vi "realgas Soave 2.1.vi"(0 "Stoffmenge H2 [mol]":dbl, 1 "Stoffmenge CH4 [mol]":dbl, 2 "Stoffmenge C2H2 [mol]":dbl, 3 "Stoffmenge O2 [mol]":dbl, 4 "Stoffmenge N2 [mol]":dbl, 5 "T [K]":dbl, 8 "1. Befüllschritt":u16(ring) items=["H2", "CH4", "C2H2", "O2", "N2"], 9 "4. Befüllschritt":u16(ring) items=["H2", "CH4", "C2H2", "O2", "N2"], 10 "2. Befüllschritt":u16(ring) items=["H2", "CH4", "C2H2", "O2", "N2"], 11 "5. Befüllschritt":u16(ring) items=["H2", "CH4", "C2H2", "O2", "N2"], 12 "3. Befüllschritt":u16(ring) items=["H2", "CH4", "C2H2", "O2", "N2"]) -> (20 "Druck [bar]":ext[](array[numeric]))   [LabVIEW 2009]
uses:
  <vilib>/express/express arith-compare/Formula/XNode/ExpressFormulaBlockNode.xnode
  <vilib>/Analysis/NI_AALBase.lvlib
  <vilib>/Analysis/baseanly.llb/Real Outer Product.vi
  <vilib>/Analysis/baseanly.llb/Real Dot Product.vi
panel:
  in  "Stoffwerte der Gase":cluster{"Tabellenwerte":dbl[]}[](array[cluster])
  in  "Kammervolumen [m^3]":dbl
  # "Befüllreihenfolge"
  # "nach 1. Schritt"
  # "nach 2. Schritt"
  # "nach 3. Schritt"
  # "nach 4. Schritt"
  # "nach 5. Schritt"
  # "p,c [Pa]"
  # "Azentischer Wert"
  # "T,c [K]"
  # "H2"
  # "CH4"
  # "C2H2"
  # "O2"
  # "N2"
  # "CO2"
  # "H2O"
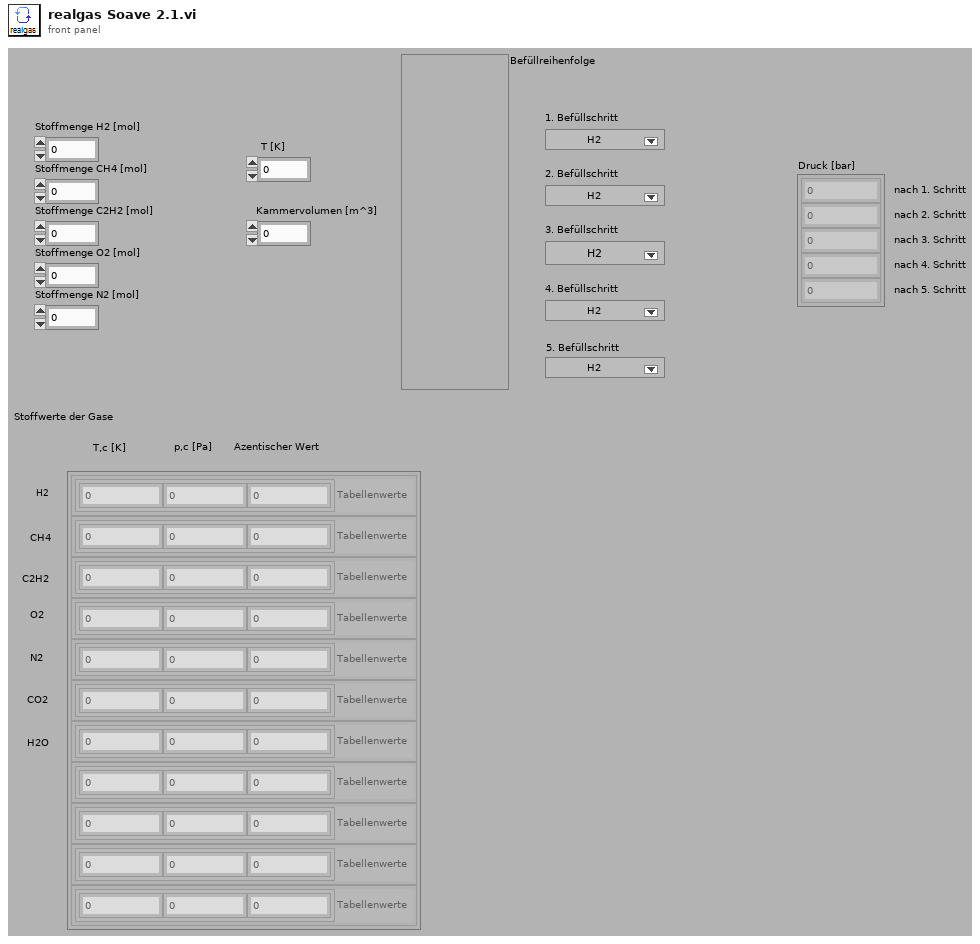
[diagram p1: front panel]
types:
  T1 = typedef "NI_Matrix.lvlib/RealMatrix.ctl" = dbl[][]
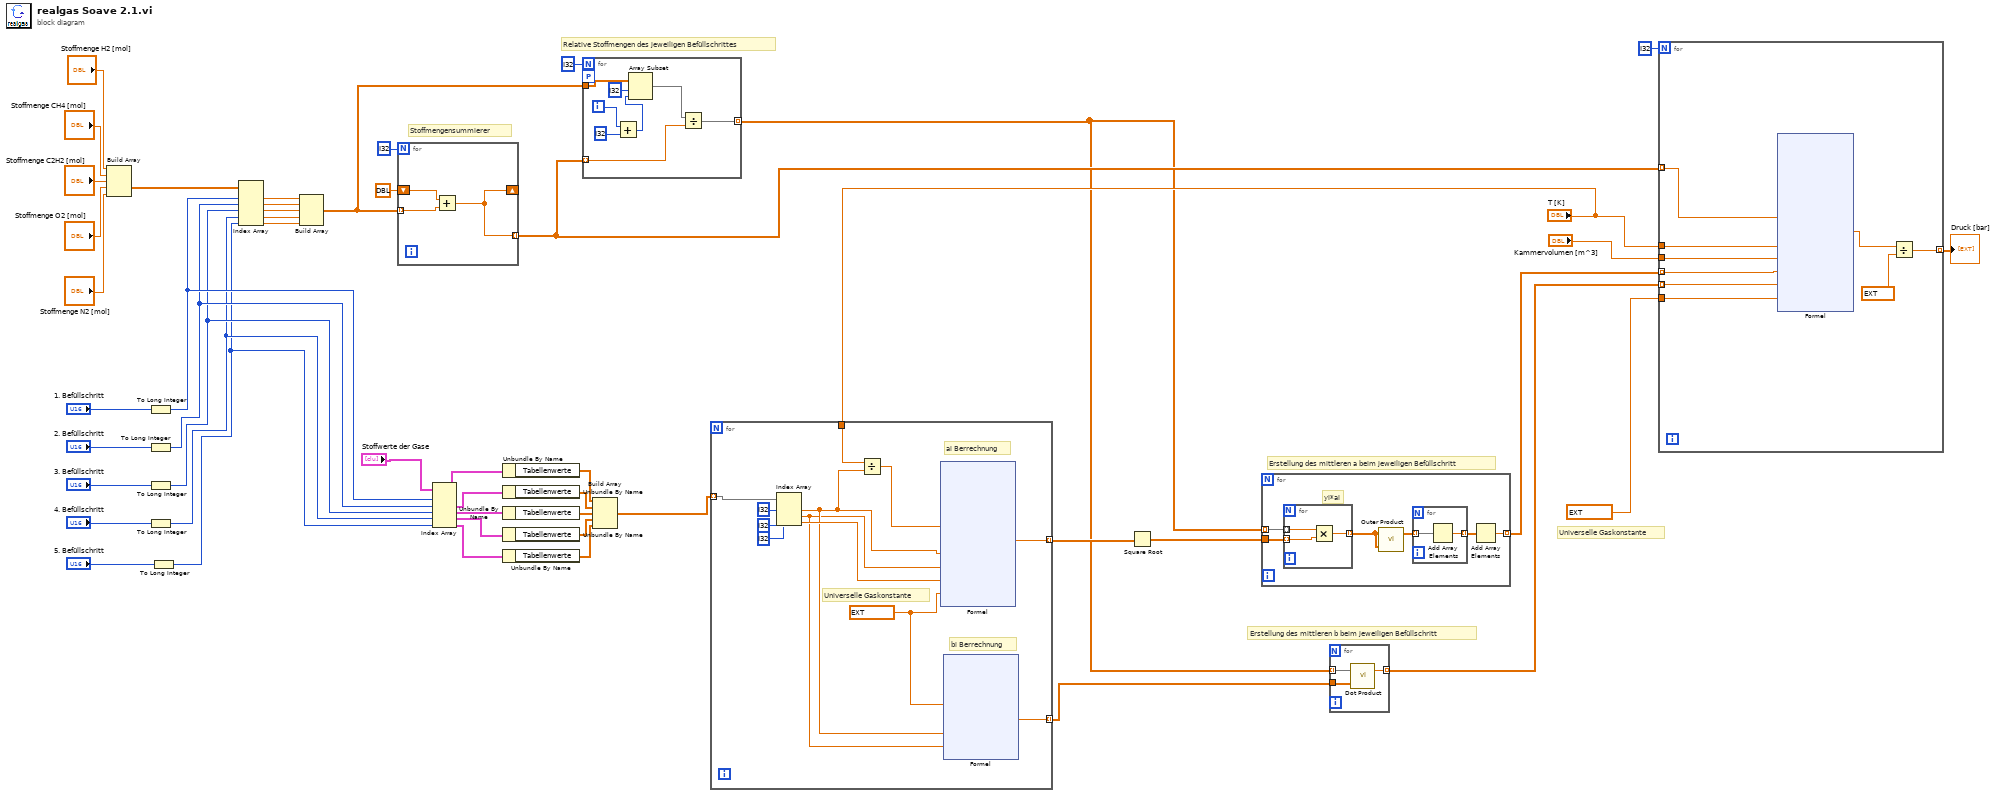
[diagram p0: block diagram]
diagram:
  # "Erstellung des mittleren b beim jeweiligen Befüllschritt"
  # "Relative Stoffmengen des jeweiligen Befüllschrittes"
  # "Stoffmengensummierer"
  # "Erstellung des mittleren a beim jeweiligen Befüllschritt"
  # "Universelle Gaskonstante"
  n1 = Build Array("Stoffmenge H2 [mol]", "Stoffmenge CH4 [mol]", "Stoffmenge C2H2 [mol]", "Stoffmenge O2 [mol]", "Stoffmenge N2 [mol]") -> (w39:dbl[])
  n2 = To Long Integer(number="1. Befüllschritt") -> (32bit integer=w26:i32)
  n3 = To Long Integer(number="2. Befüllschritt") -> (32bit integer=w25:i32)
  n4 = To Long Integer(number="3. Befüllschritt") -> (32bit integer=w24:i32)
  n5 = To Long Integer(number="4. Befüllschritt") -> (32bit integer=w23:i32)
  n6 = To Long Integer(number="5. Befüllschritt") -> (32bit integer=w22:i32)
  n7 = Index Array(array=w39, index #1=w26, index #2=w25, index #3=w24, index #4=w23, index #5=w22) -> (element #1=w38:dbl, element #2=w37:dbl, element #3=w36:dbl, element #4=w35:dbl, element #5=w34:dbl)
  n8 = Build Array(w38, w37, w36, w35, w34) -> (w10:dbl[])
  n9 = for {
    N: i32 ? -> [_]
    tunnel: w10 -> [w52] mode=indexing
    shift-right: [w50] -> _
    shift-left: dbl ? -> [w51]
    tunnel: [w50] -> w5 mode=indexing
    n10 = Add(x=w51, y=w52) -> (x+y=w50:dbl)
  }
  n11 = Index Array(array="Stoffwerte der Gase", index #1=w26, index #2=w25, index #3=w24, index #4=w23, index #5=w22) -> (element #1=w27:cluster{"Tabellenwerte":dbl[]}, element #2=w21:cluster{"Tabellenwerte":dbl[]}, element #3=w20:cluster{"Tabellenwerte":dbl[]}, element #4=w19:cluster{"Tabellenwerte":dbl[]}, element #5=w18:cluster{"Tabellenwerte":dbl[]})
  n12 = Unbundle By Name(w27) -> ("Tabellenwerte"=w17:dbl[])
  n13 = Unbundle By Name(w21) -> ("Tabellenwerte"=w16:dbl[])
  n14 = Unbundle By Name(w20) -> ("Tabellenwerte"=w15:dbl[])
  n15 = Unbundle By Name(w19) -> ("Tabellenwerte"=w14:dbl[])
  n16 = Unbundle By Name(w18) -> ("Tabellenwerte"=w13:dbl[])
  n17 = for {
    N: i32 ? -> [_]
    tunnel: w10 -> [w60]
    tunnel: w5 -> [w55] mode=indexing
    workers-P: _ -> [_]
    tunnel: [w53] -> w3 mode=indexing
    i -> [w58]
    n18 = Add(x=w58, y=i32 ?) -> (x+y=w56:i32)
    n19 = Array Subset(array=w60, index=i32 ? ("Index"), length=w56) -> (w54:dbl[])
    n20 = Divide(x=w54, y=w55) -> (x/y=w53:dbl[])
  }
  n21 = Build Array(w17, w16, w15, w14, w13) -> (w12:dbl[][])
  n22 = for {
    tunnel: w12 -> [w72] mode=indexing
    tunnel: "T [K]" -> [w68]
    tunnel: [w65] -> w7 mode=indexing
    tunnel: [w61] -> w4 mode=indexing
    w64 = ext ? ("Wert")
    # "bi Berrechnung"
    # "ai Berrechnung"
    # "Universelle Gaskonstante"
    n23 = Index Array(array=w72, index #1=i32 ? ("Index"), index #2=i32 ? ("Index"), index #3=i32 ? ("Index")) -> (element #1=w63:dbl, element #2=w62:dbl, element #3=w66:dbl)
    n24 = Divide(x=w68, y=w63) -> (x/y=w67:dbl)
    n25 = xnode "Formel"("Tr"=w67, "Tc"=w63, "pc"=w62, "Omega"=w66, "R"=w64) -> ("Ergebnis"=w65:ext)  [unwired: 1 in, 1 out]
    n26 = xnode "Formel"("R"=w64, "Tc"=w63, "pc"=w62) -> ("Ergebnis"=w61:ext)  [unwired: 1 in, 1 out]
  }
  n27 = Square Root(x=w7) -> (sqrt(x)=w6:ext[])
  n28 = for {
    tunnel: [w104] -> w2 mode=indexing
    tunnel: w6 -> [w102]
    tunnel: w3 -> [w103] mode=indexing
    # "yi*ai"
    n29 = for {
      tunnel: w102 -> [w109] mode=indexing
      tunnel: [w108] -> w101 mode=indexing
      tunnel: w103 -> [w107] mode=indexing
      n30 = Multiply(x=w107, y=w109) -> (x*y=w108:ext)
    }
    n31 = call-poly <vilib>:"Outer Product.vi"("Y Vector"=w101, "X Vector"=w101) -> ("Outer Product"=w106:T1)  [unwired: 1 out]
    n32 = for {
      tunnel: w106 -> [w111] mode=indexing
      tunnel: [w110] -> w105 mode=indexing
      n33 = Add Array Elements(numeric array=w111) -> (sum=w110:dbl)
    }
    n34 = Add Array Elements(numeric array=w105) -> (sum=w104:dbl)
  }
  n35 = for {
    tunnel: w3 -> [w113] mode=indexing
    tunnel: [w114] -> w1 mode=indexing
    tunnel: w4 -> [w112]
    n36 = call-poly <vilib>:"Dot Product.vi"("Y Vector"=w112, "X Vector"=w113) -> ("X * Y"=w114:dbl)  [unwired: 1 out]
  }
  n37 = for {
    N: i32 ? -> [_]
    tunnel: "Kammervolumen [m^3]" -> [w123]
    tunnel: ext ? ("Wert") -> [w122]
    tunnel: "T [K]" -> [w121]
    tunnel: w5 -> [w120] mode=indexing
    tunnel: [w117] -> w8 mode=indexing
    tunnel: w2 -> [w116] mode=indexing
    tunnel: w1 -> [w115] mode=indexing
    n38 = xnode "Formel"("n"=w120, "T"=w121, "V"=w123, "a"=w116, "b"=w115, "R"=w122) -> ("Ergebnis"=w119:ext)  [unwired: 1 in, 1 out]
    n39 = Divide(x=w119, y=ext ?) -> (x/y=w117:ext)
  }
  "Druck [bar]" <- w8
